vi "Get Add States Terminals.vi"(8 "error in (no error)":errorcluster, 11 "Add State(s) to Queue ref":refnum<vi>) -> (0 "error out":errorcluster, 1 "States Out":refnum<vi>, 2 "State(s) at Back (\"\")":refnum<vi>, 3 "State(s) in (\"\")":refnum<vi>, 5 "State(s) in Front (\"\")":refnum<vi>)   [LabVIEW 2013, in "JKI State Machine API.lvlib" / "JKI SM.lvclass"]
uses:
  JKI SM.lvclass
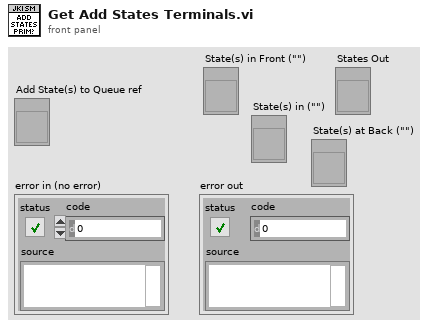
[diagram p1: front panel]
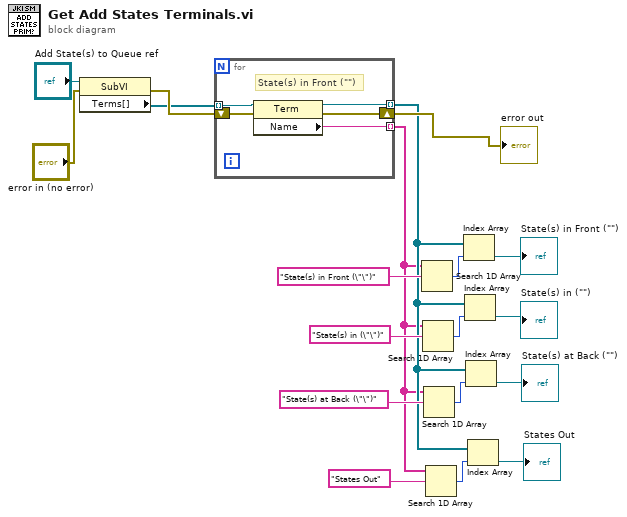
[diagram p0: block diagram]
diagram:
  n1 = property class="SubVI"(reference="Add State(s) to Queue ref", error in="error in (no error)") -> (error out=w18:errorcluster, "Terms[]"=w16:refnum<vi>[])  [unwired: 1 out]
  n2 = for {
    tunnel: w16 -> [w24] mode=indexing
    shift-right: [w22] -> w15
    shift-left: w18 -> [w23]
    tunnel: [w21] -> w1 mode=indexing
    tunnel: [w20] -> w2 mode=indexing
    # "State(s) in Front (\"\")"
    n3 = property class="Term"(reference=w24, error in=w23) -> (reference out=w20:refnum<vi>, error out=w22:errorcluster, "Name"=w21:string)
  }
  "error out" <- w15
  n4 = Search 1D Array(1D array=w1, element="State(s) in Front (\"\")" ("Name")) -> (index of element=w14:i32)  [unwired: 1 in]
  n5 = Search 1D Array(1D array=w1, element="State(s) in (\"\")" ("Name")) -> (index of element=w11:i32)  [unwired: 1 in]
  n6 = Search 1D Array(1D array=w1, element="State(s) at Back (\"\")" ("Name")) -> (index of element=w10:i32)  [unwired: 1 in]
  n7 = Search 1D Array(1D array=w1, element="States Out" ("Name")) -> (index of element=w3:i32)  [unwired: 1 in]
  n8 = Index Array(array=w2, index=w14) -> (element=→"State(s) in Front (\"\")":refnum<vi>)
  n9 = Index Array(array=w2, index=w11) -> (element=→"State(s) in (\"\")":refnum<vi>)
  n10 = Index Array(array=w2, index=w10) -> (element=→"State(s) at Back (\"\")":refnum<vi>)
  n11 = Index Array(array=w2, index=w3) -> (element=→"States Out":refnum<vi>)
